vi "Save.vi"() -> ()   [LabVIEW 2021, in "Main.lvlib"]
doc: "This VI, is used saving the information to a log file.\n1. First window opens. If the user clicks cancel the default log file will be picked. If wrong file is picked, dialog window will be generated. \n2. If there is missing information dialog window will be generated. \n3. Click save to save to the log file.\n4. Click Exit to exit the VI"
uses:
  Main.lvlib
  Tipski Definicii/Save_Sostojbi.ctl
  Polymorphic/Enq_Save_QMH.vi
  Polymorphic/DeQ_Save_QMH.vi
  subVIS/Main_Programs_SubVIs.lvlib
  Polymorphic/Queues.lvlib
panel:
  in  "Exit Progam":bool
  out "Picked Path":path
  in  "Surname":string
  in  "Save Log":bool
  in  "Instrument":string
  in  "Lab":string
  in  "Name":string
  # "The default path is: This VI/subVIS/Log.csv"
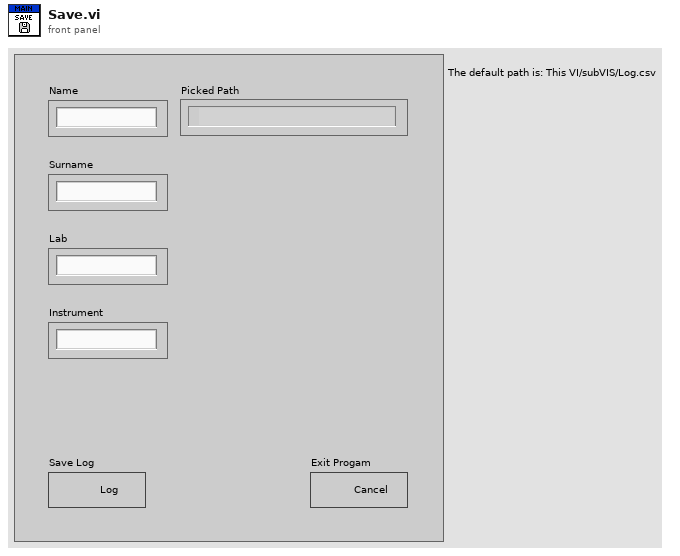
[diagram p1: front panel]
types:
  T1 = cluster{"Main Queue":refnum<queue>, "ER Refnum":refnum<event-registration>, "User Event":refnum<user-event>}
  T2 = typedef "Save_program_queues.ctl" = cluster{"Main Queue":refnum<queue>, "ER Refnum":refnum<event-registration>, "User Event":refnum<user-event>}
  T3 = typedef "Save_Sostojbi.ctl" = enum16{"Init", "Generate Message", "Pick Path", "Save", "End"}
  T4 = enum32{"Invalid", "Standard", "Closed", "Hidden", "Minimized", "Maximized"}
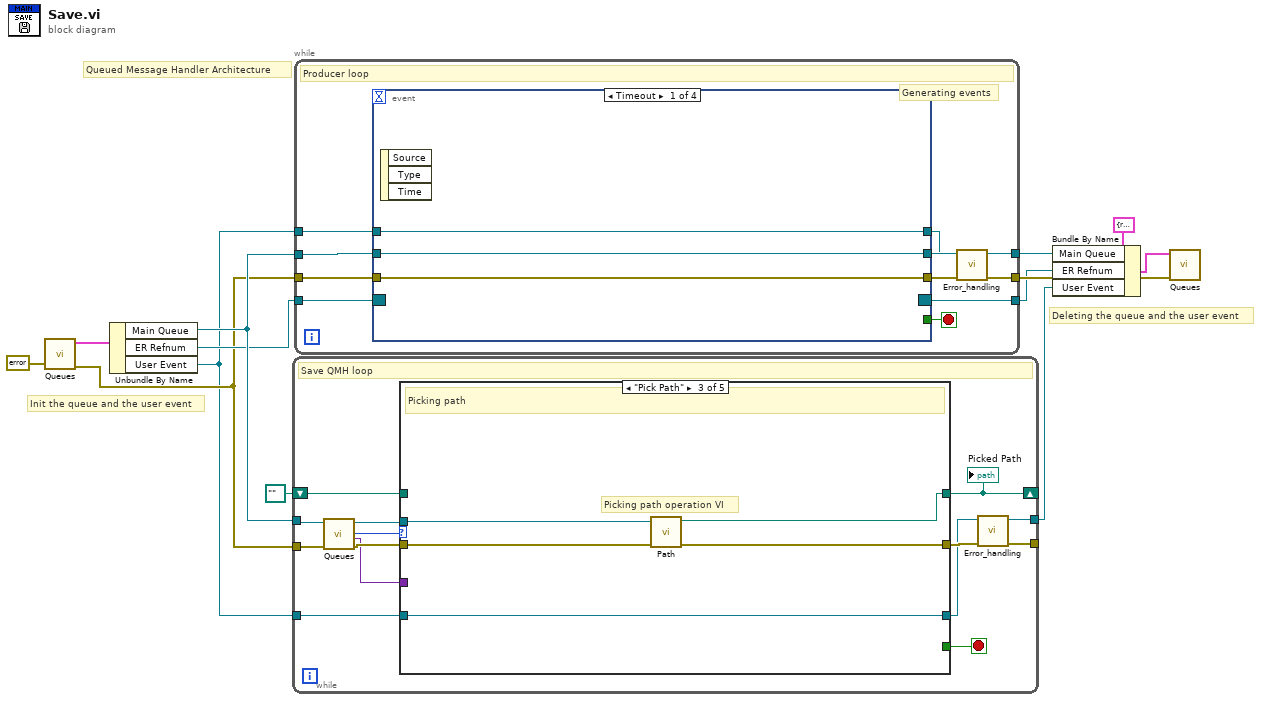
[diagram p0: block diagram]
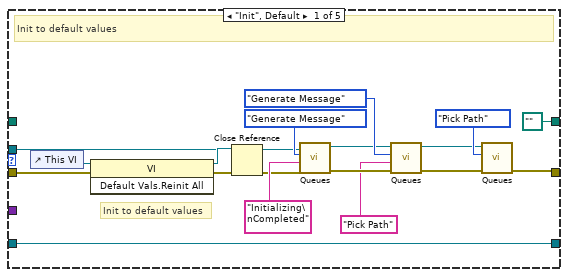
[diagram p2: hidden frame]
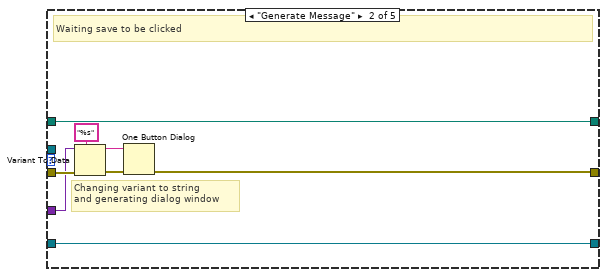
[diagram p3: hidden frame]
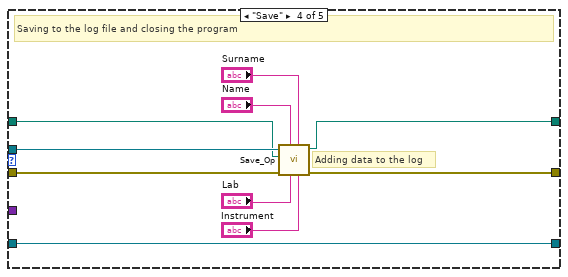
[diagram p4: hidden frame]
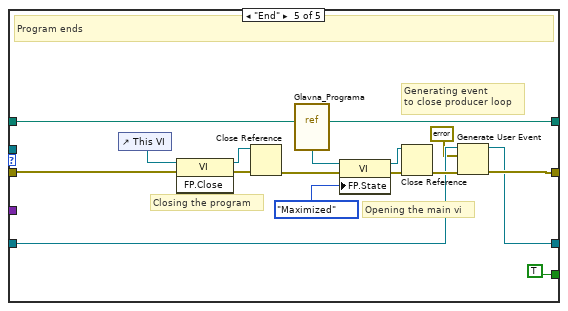
[diagram p5: hidden frame]
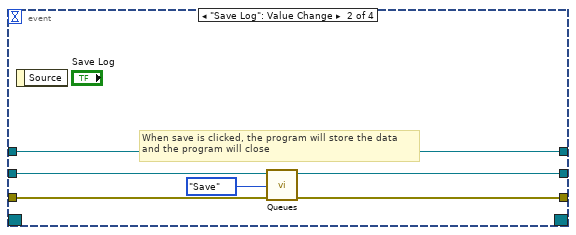
[diagram p6: hidden frame]
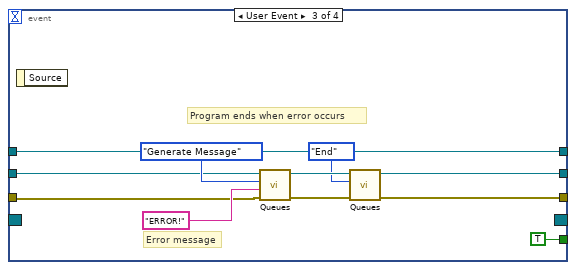
[diagram p7: hidden frame]
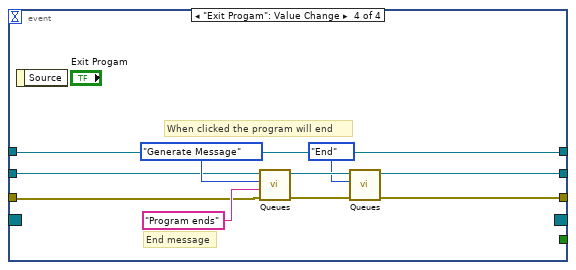
[diagram p8: hidden frame]
diagram:
  # "Deleting the queue and the user event"
  # "Queued Message Handler Architecture"
  # "Init the queue and the user event"
  n1 = call-poly "Queues.vi"("Error In"=errorcluster {"status"=FALSE, "code"=0, "source"=""}) -> ("Error Out"=w8:errorcluster, "Queue Cluster"=w11:T2)  [unwired: 9 in]
  n2 = Unbundle By Name(w11) -> ("Main Queue"=w10:refnum<queue>, "ER Refnum"=w9:refnum<event-registration>, "User Event"=w1:refnum<user-event>)
  n3 = while {
    tunnel: w8 -> [w19]
    tunnel: w10 -> [w18]
    shift-right: [w26] -> _
    shift-left: path "" ("appended path") -> [w25]
    tunnel: w1 -> [w24]
    tunnel: [w22] -> _
    tunnel: [w21] -> w3
    stop <- w27 stop-if-true
    # "Save QMH loop"
    n4 = call-poly "Queues.vi"("Error In"=w19, "Queue In"=w18) -> ("Error Out"=w16:errorcluster, "Message"=w14:variant, "Instruction"=w15:T3, "Queue Out"=w17:refnum<queue>)  [unwired: 6 in]
    n5 = case shown="\"Pick Path\"" w15 {
      tunnel: w17 -> [w31 _ w53 w66 _]
      tunnel: w16 -> [w45 w52 w57 w67 w73]
      tunnel: [w28 w48 w55 w65 w71] -> w23
      tunnel: [_ _ _ _ TRUE] -> w27
      tunnel: w14 -> [_ w51 _ _ _]
      tunnel: [path "" ("appended path") w46 w56 w62 w83] -> w26
      tunnel: w25 -> [_ w46 _ w63 w83]
      tunnel: w24 -> [w41 w47 w54 w64 w70]
      tunnel: [w41 w47 w54 w64 w69] -> w20
      frame "Init", Default {
        # "Init to default values"
        # "Init to default values"
        n6 = control-ref of="This VI"() -> (w44:refnum<vi>)
        n7 = invoke class="VI" method="Default Vals.Reinit All"(reference=w44, error in=w45) -> (reference out=w42:refnum<vi>, error out=w43:errorcluster)  [unwired: 1 in, 1 out]
        n8 = Close Reference(reference=w42, error in (no error)=w43) -> (error out=w32:errorcluster)
        n9 = call-poly "Queues.vi"("Error In"=w32, "Message"="Initializing\nCompleted", "Instruction"=Save_Sostojbi."Generate Message", "Queue In"=w31) -> ("Error Out"=w38:errorcluster, "Queue Out"=w30:refnum<queue>)  [unwired: 6 in]
        n10 = call-poly "Queues.vi"("Error In"=w38, "Message"="Pick Path", "Instruction"=Save_Sostojbi."Generate Message", "Queue In"=w30) -> ("Error Out"=w39:errorcluster, "Queue Out"=w29:refnum<queue>)  [unwired: 6 in]
        n11 = call-poly "Queues.vi"("Error In"=w39, "Instruction"=Save_Sostojbi."Pick Path", "Queue In"=w29) -> ("Error Out"=w28:errorcluster)  [unwired: 7 in, 1 out]
      }
      frame "Generate Message" {
        # "Changing variant to string \nand generating dialog window"
        # "Waiting save to be clicked"
        n12 = Variant To Data(error in=w52, type="%s", Variant=w51) -> (data=w49:string, error out=w48:errorcluster)
        n13 = One Button Dialog(message=w49) -> ()  [unwired: 1 in, 1 out]
      }
      frame "Pick Path" {
        # "Picking path operation VI"
        # "Picking path"
        n14 = call "Path.vi"("Error In"=w57, "Queue in"=w53) -> ("Error Out"=w55:errorcluster, "Output Path"=w56:path)  [unwired: 8 in]
      }
      frame "Save" {
        # "Adding data to the log"
        # "Saving to the log file and closing the program"
        n15 = call "Save_Op.vi"("Instrument"="Instrument", "Surname"="Surname", "Lab"="Lab", "Name"="Name", "Error In"=w67, "Path In"=w63, "Queue in"=w66) -> ("Error Out"=w65:errorcluster, "Path Out"=w62:path)  [unwired: 3 in]
      }
      frame "End" {
        # "Generating event\nto close producer loop"
        # "Opening the main vi"
        # "Closing the program"
        # "Program ends"
        n16 = control-ref of="This VI"() -> (w74:refnum<vi>)
        n17 = invoke class="VI" method="FP.Close"(reference=w74, error in=w73) -> (reference out=w76:refnum<vi>, error out=w75:errorcluster)  [unwired: 1 in, 1 out]
        n18 = Close Reference(reference=w76, error in (no error)=w75) -> (error out=w77:errorcluster)
        n19 = vi-ref "Glavna_Programa.vi"() -> (w78:refnum<vi>)
        n20 = property class="VI"(reference=w78, error in=w77, "FP.State"=T4."Maximized" ("Front Panel Window:State")) -> (reference out=w81:refnum<vi>, error out=w80:errorcluster)
        n21 = Close Reference(reference=w81, error in (no error)=w80) -> (error out=w72:errorcluster)
        n22 = Generate User Event(user event=w70, event data cluster=errorcluster {"status"=FALSE, "code"=0, "source"=""} ("event data"), error in=w72) -> (user event out=w69:refnum<user-event>, error out=w71:errorcluster)  [unwired: 1 in]
      }
    }
    "Picked Path" <- w26
    n23 = call "Error_handling.vi"("Error In"=w23, "User Event in"=w20) -> ("Error Out"=w22:errorcluster, "User Event out"=w21:refnum<user-event>)  [unwired: 8 in]
  }
  n24 = while {
    tunnel: w10 -> [w93]
    tunnel: w8 -> [w92]
    tunnel: [w91] -> w5
    tunnel: [w86] -> w7
    tunnel: [w90] -> w4
    tunnel: w9 -> [w89]
    tunnel: w1 -> [w85]
    stop <- w88 stop-if-true
    # "Generating events"
    # "Producer loop"
    n25 = event shown="[0] Timeout" {
      selector: w89 -> [_ _ _ _]
      dyn-events: [_ _ _ _] -> w90
      timeout: _ -> [_ _ _ _]
      tunnel: w93 -> [w96 w101 w106 w116]
      tunnel: w92 -> [w95 w102 w107 w118]
      tunnel: [w96 w100 w105 w115] -> w91
      tunnel: [w95 w99 w104 w117] -> w87
      tunnel: [_ _ TRUE _] -> w88
      tunnel: w85 -> [w94 w97 w103 w114]
      tunnel: [w94 w97 w103 w114] -> w84
      event Timeout {
        n26 = event-data() -> ()  [unwired: 1 in, 3 out]
      }
      event "Save Log": Value Change {
        # "When save is clicked, the program will store the data\nand the program will close"
        n27 = event-data() -> ()  [unwired: 1 in, 1 out]
        n28 = call-poly "Queues.vi"("Error In"=w102, "Instruction"=Save_Sostojbi."Save", "Queue In"=w101) -> ("Error Out"=w99:errorcluster, "Queue Out"=w100:refnum<queue>)  [unwired: 7 in]
      }
      event User Event {
        # "Error message"
        # "Program ends when error occurs"
        n29 = event-data() -> ()  [unwired: 1 in, 1 out]
        n30 = call-poly "Queues.vi"("Error In"=w107, "Message"="ERROR!", "Instruction"=Save_Sostojbi."Generate Message", "Queue In"=w106) -> ("Error Out"=w111:errorcluster, "Queue Out"=w112:refnum<queue>)  [unwired: 6 in]
        n31 = call-poly "Queues.vi"("Error In"=w111, "Instruction"=Save_Sostojbi."End", "Queue In"=w112) -> ("Error Out"=w104:errorcluster, "Queue Out"=w105:refnum<queue>)  [unwired: 7 in]
      }
      event "Exit Progam": Value Change {
        # "End message"
        # "When clicked the program will end"
        n32 = event-data() -> ()  [unwired: 1 in, 1 out]
        n33 = call-poly "Queues.vi"("Error In"=w118, "Message"="Program ends", "Instruction"=Save_Sostojbi."Generate Message", "Queue In"=w116) -> ("Error Out"=w122:errorcluster, "Queue Out"=w123:refnum<queue>)  [unwired: 6 in]
        n34 = call-poly "Queues.vi"("Error In"=w122, "Instruction"=Save_Sostojbi."End", "Queue In"=w123) -> ("Error Out"=w117:errorcluster, "Queue Out"=w115:refnum<queue>)  [unwired: 7 in]
      }
    }
    n35 = call "Error_handling.vi"("Error In"=w87, "User Event in"=w84) -> ("Error Out"=w86:errorcluster)  [unwired: 8 in, 1 out]
  }
  n36 = Bundle By Name(cluster=T1 {"Main Queue"=refnum, "ER Refnum"=refnum, "User Event"=refnum} ("Queue Cluster"), "Main Queue"=w5, "ER Refnum"=w4, "User Event"=w3) -> (w2:T1)
  n37 = call-poly "Queues.vi"("Error In"=w7, "Queue Cluster"=w2) -> ()  [unwired: 10 in]
